vi "GVChroms.vi"() -> ()   [LabVIEW 2017]
panel:
  out "ECD2Chrom":dbl[](array[numeric])
  out "ECD1Chrom":dbl[](array[numeric])
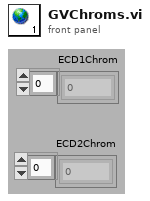
[diagram p1: front panel]
diagram:
